vi "Get All Songs.vi"(8 "error in (no error)":errorcluster, 11 "MusicLibrary in":refnum<class "MusicLibrary.lvclass">) -> (0 "error out":errorcluster, 2 "Songs":refnum<class "Song.lvclass">[](array[class]), 3 "MusicLibrary out":refnum<class "MusicLibrary.lvclass">)   [LabVIEW 2015, in "MusicLibrary.lvclass"]
uses:
  MusicLibrary.lvclass
  Song/Song.lvclass
  MusicElementLibrary.lvclass/MusicElementLibrary.ctl
  SongLibrary/SongLibrary.lvclass
  Album/Album.lvclass/Album.ctl
  MusicElement.lvclass
  MusicElementLibrary.lvclass
  Album/Album.lvclass
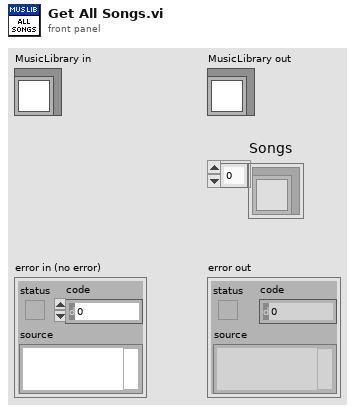
[diagram p1: front panel]
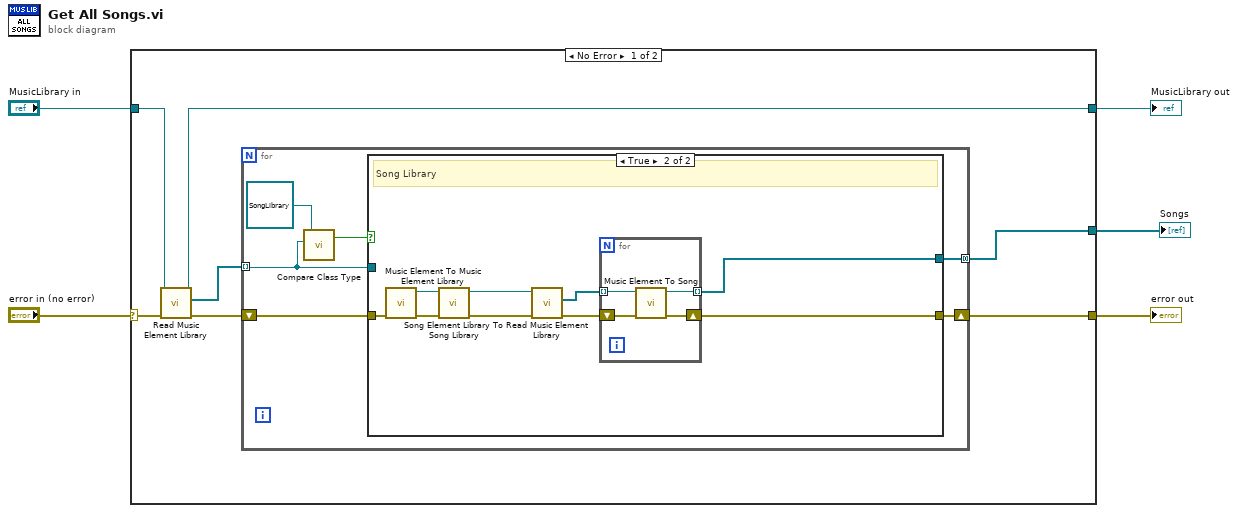
[diagram p0: block diagram]
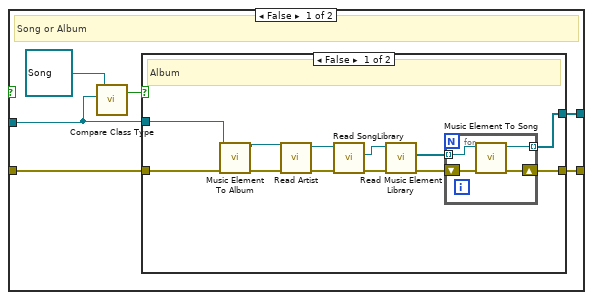
[diagram p2: hidden frame]
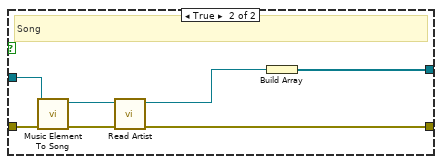
[diagram p3: hidden frame]
diagram:
  n1 = case shown="No Error" "error in (no error)" {
    selector: "error in (no error)" -> [w12 w62]
    tunnel: [w7 w62] -> w4
    tunnel: [w9 w61] -> w2
    tunnel: "MusicLibrary in" -> [w10 w61]
    tunnel: [w6 _] -> w1
    frame No Error {
      n2 = call "Read Music Element Library.vi"("error in (no error)"=w12, "MusicElementLibrary in"=w10) -> ("error out"=w11:errorcluster, "Music Element Library"=w8:refnum<class "MusicElement.lvclass">[], "MusicElementLibrary out"=w9:refnum<class "MusicLibrary.lvclass">)  [unwired: 7 in]
      n3 = for {
        shift-right: [w18] -> w7
        shift-left: w11 -> [w13]
        tunnel: w8 -> [w15] mode=indexing
        tunnel: [w17] -> w6 mode=concatenating
        n4 = call "Compare Class Type.vi"("MusicElement Check"=w15, "MusicElement in"=refnum<class "SongLibrary.lvclass"> refnum ("SongLibrary out")) -> ("Same Class Type?"=w14:bool)  [unwired: 3 in]
        n5 = case shown="True" w14 {
          tunnel: [w24 w53] -> w18
          tunnel: [w23 w54] -> w17
          tunnel: w15 -> [w19 _]
          tunnel: w13 -> [w21 w50]
          frame False {
            # "Song or Album"
            n6 = call "Compare Class Type.vi"("MusicElement Check"=w19, "MusicElement in"=refnum<class "Song.lvclass"> refnum ("Song out")) -> ("Same Class Type?"=w22:bool)  [unwired: 3 in]
            n7 = case shown="False" w22 {
              tunnel: [w33 w47] -> w24
              tunnel: [w26 w46] -> w23
              tunnel: w19 -> [w35 w43]
              tunnel: w21 -> [w25 w44]
              frame False {
                # "Album"
                n8 = call "Music Element To Album.vi"("error in (no error)"=w25, "MusicElement"=w35) -> ("error out"=w36:errorcluster, "Album"=w34:refnum<class "Album.lvclass">)  [unwired: 8 in]
                n9 = call "Read Artist.vi"("error in (no error)"=w36, "Album in"=w34) -> ("error out"=w32:errorcluster, "Album out"=w31:refnum<class "Album.lvclass">)  [unwired: 7 in, 1 out]
                n10 = call "Read SongLibrary.vi"("error in (no error)"=w32, "Album in"=w31) -> ("error out"=w30:errorcluster, "SongLibrary.lvclass"=w29:refnum<class "SongLibrary.lvclass">)  [unwired: 7 in, 1 out]
                n11 = call "Read Music Element Library.vi"("error in (no error)"=w30, "MusicElementLibrary in"=w29) -> ("error out"=w27:errorcluster, "Music Element Library"=w28:refnum<class "MusicElement.lvclass">[])  [unwired: 7 in, 1 out]
                n12 = for {
                  shift-right: [w39] -> w33
                  shift-left: w27 -> [w40]
                  tunnel: w28 -> [w38] mode=indexing
                  tunnel: [w37] -> w26 mode=indexing
                  n13 = call "Music Element To Song.vi"("error in (no error)"=w40, "MusicElement"=w38) -> ("error out"=w39:errorcluster, "Song out"=w37:refnum<class "Song.lvclass">)  [unwired: 8 in]
                }
              }
              frame True {
                # "Song"
                n14 = call "Music Element To Song.vi"("error in (no error)"=w44, "MusicElement"=w43) -> ("error out"=w41:errorcluster, "Song out"=w42:refnum<class "Song.lvclass">)  [unwired: 8 in]
                n15 = call "Read Artist.vi"("error in (no error)"=w41, "Song in"=w42) -> ("error out"=w47:errorcluster, "Song out"=w45:refnum<class "Song.lvclass">)  [unwired: 7 in, 1 out]
                n16 = Build Array(w45) -> (w46:refnum<class "Song.lvclass">[])
              }
            }
          }
          frame True {
            # "Song Library"
            n17 = call "Music Element To Music Element Library.vi"("error in (no error)"=w50) -> ("error out"=w51:errorcluster, "MusicElementLibrary out"=w52:refnum<class "MusicElementLibrary.lvclass">)  [unwired: 9 in]
            n18 = call "Song Element Library To Song Library.vi"("error in (no error)"=w51, "MusicElementLibrary"=w52) -> ("error out"=w49:errorcluster, "SongLibrary out"=w48:refnum<class "SongLibrary.lvclass">)  [unwired: 8 in]
            n19 = call "Read Music Element Library.vi"("error in (no error)"=w49, "MusicElementLibrary in"=w48) -> ("error out"=w56:errorcluster, "Music Element Library"=w55:refnum<class "MusicElement.lvclass">[])  [unwired: 7 in, 1 out]
            n20 = for {
              shift-right: [w59] -> w53
              shift-left: w56 -> [w60]
              tunnel: w55 -> [w58] mode=indexing
              tunnel: [w57] -> w54 mode=indexing
              n21 = call "Music Element To Song.vi"("error in (no error)"=w60, "MusicElement"=w58) -> ("error out"=w59:errorcluster, "Song out"=w57:refnum<class "Song.lvclass">)  [unwired: 8 in]
            }
          }
        }
      }
    }
    frame Error {
    }
  }
  "error out" <- w4
  "MusicLibrary out" <- w2
  "Songs" <- w1
